vi "Live Imaging Window.vi"() -> ()   [LabVIEW 2020]
uses:
  Typedefs/Channel Selector.ctl
  SubVIs/Typedefs/Live window-ctrl refs.ctl
  Typedefs/Image display ref.ctl
  Typedefs/Left-Right enum.ctl
  Global Variables/General Globals.vi
  Globals/gl_Windows Ctrl refs.vi
panel:
  in  "Grid Visible":bool
  in  "Grid Lines":u32=2 min=2 max=10 step=1
  in  "Boolean":bool=TRUE
  in  "Pal":u32(ring) items=["Grayscale", "Binary", "Gradient", "Rainbow", "Temperature", "User Defined"]
  out "Running":bool
  out "Stop (ind)":bool
  in  "Snapshot Mode":bool
  out "Images received":i32
  out "Acq rate ind (Hz)":dbl format="Acquisition frame rate: %.1f fps"
  out "Refresh rate ind (Hz)":i32 format="Graph refresh rate: %.0f fps"
  in  "Right image intensity":cluster{i16, i16}(slide)={0, 2048} scale=0.0..4095.0
  in  "Right Image Palette":enum16{"Gray", "Red", "Green"}(ring) caption="Palette"
  in  "Right Channel":T1=enum."Green Channel"
  in  "Left image intensity":cluster{i16, i16}(slide)={0, 2048} scale=0.0..4095.0
  in  "Left Image Palette":enum16{"Gray", "Red", "Green"}(ring) caption="Palette"
  in  "Left Channel":T1
  in  "Sim":bool
  out "Right Image":T2(plugin-control)
  in  "Snapshot":bool
  out "Left Image":T2(plugin-control)
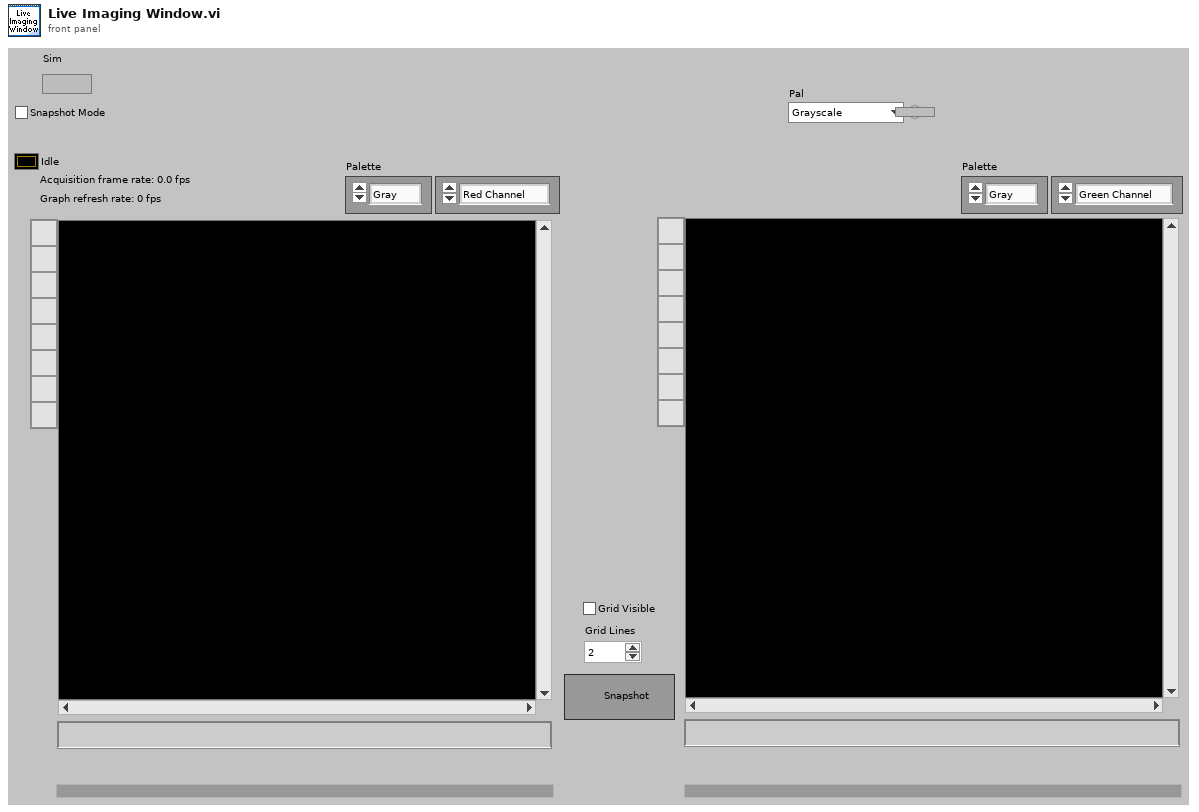
[diagram p1: front panel]
types:
  T1 = typedef "Channel Selector.ctl" = enum16{"Red Channel", "Green Channel", "Blended"}
  T2 = typedef "IMAQ Image.ctl" = refnum<image>
  T3 = typedef "Live window-ctrl refs.ctl" = cluster{"This VI":refnum<vi>, "Pane":refnum<vi>, "Show REF Image Left":refnum<vi>, "Show REF Image Right":refnum<vi>, "Snapshot":refnum<vi>, "Left Image Palette":refnum<vi>, "Right Image Palette":refnum<vi>, "Left Channel":refnum<vi>, "Right Channel":refnum<vi>, "Left image intensity":refnum<vi>, "Right image intensity":refnum<vi>, "Left Image Display":T4, "Right Image Display":T4, "Refresh rate ind (Hz)":refnum<vi>, "Acq rate ind (Hz)":refnum<vi>, "Stop (ind)":refnum<vi>}
  T4 = typedef "Image display ref.ctl" = refnum<vi>
  T5 = typedef "Live graph data queue ref.ctl" = refnum<queue>
  T6 = typedef "Left-Right enum.ctl" = enum16{"Right", "Left"}
  T7 = typedef "Live imaging queue element.ctl" = cluster{"Red channel":T2, "Green channel":T2, "Ref Red channel":T2, "Ref Green channel":T2, "Mov cor":bool}
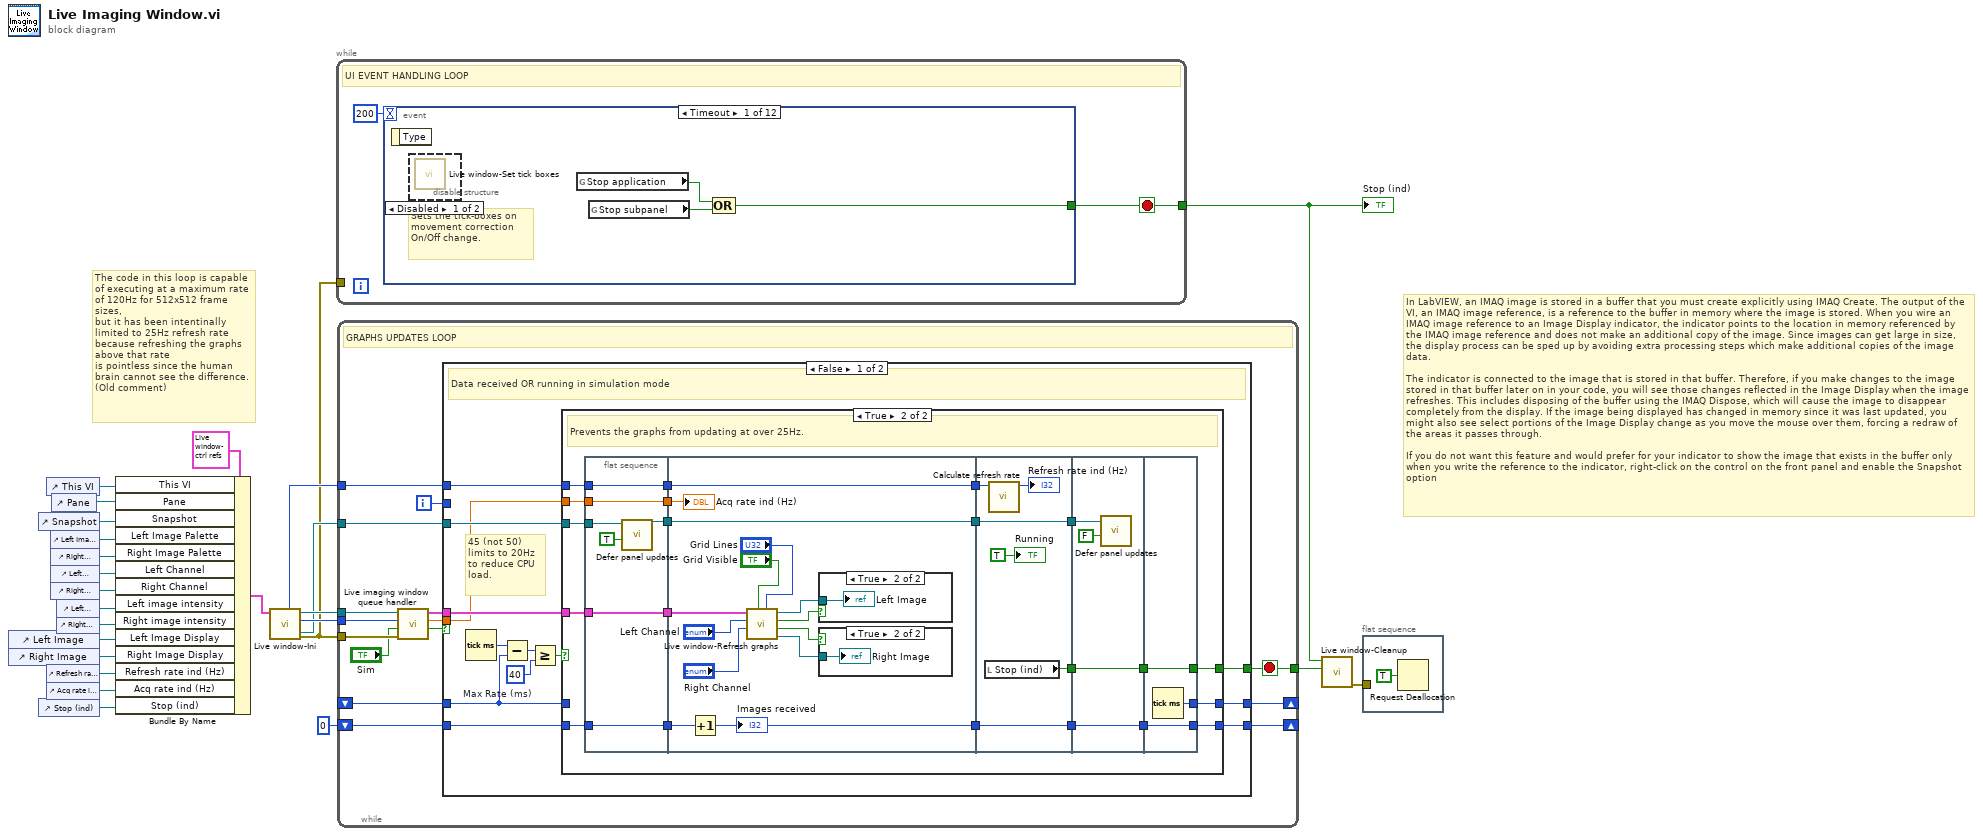
[diagram p0: block diagram]
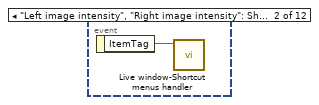
[diagram p3: hidden frame]
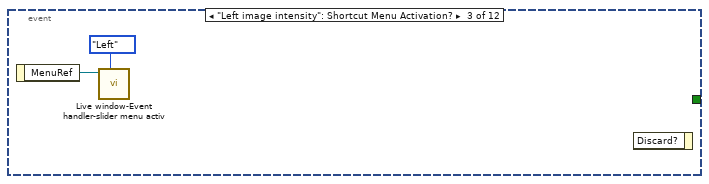
[diagram p4: hidden frame]
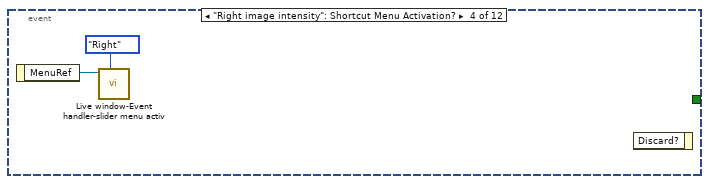
[diagram p5: hidden frame]
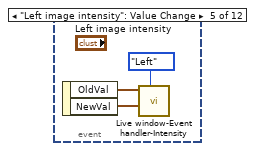
[diagram p6: hidden frame]
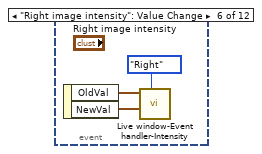
[diagram p7: hidden frame]
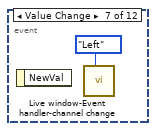
[diagram p8: hidden frame]
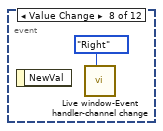
[diagram p9: hidden frame]
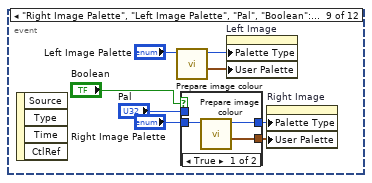
[diagram p10: hidden frame]
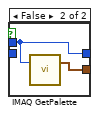
[diagram p11: hidden frame]
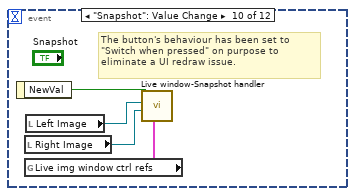
[diagram p12: hidden frame]
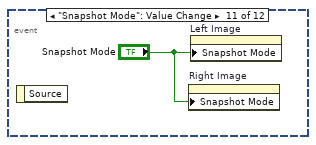
[diagram p13: hidden frame]
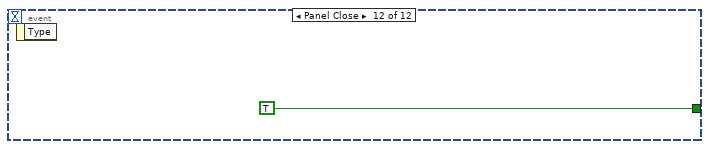
[diagram p14: hidden frame]
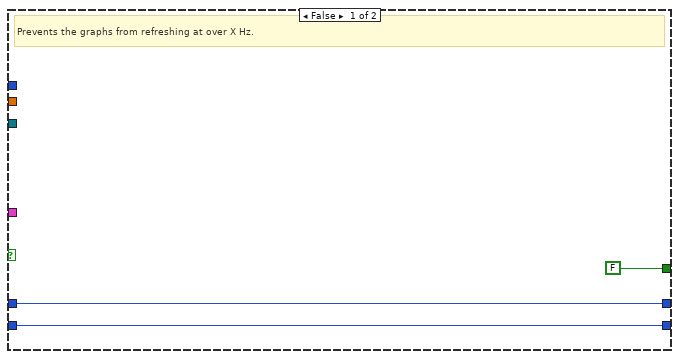
[diagram p15: hidden frame]
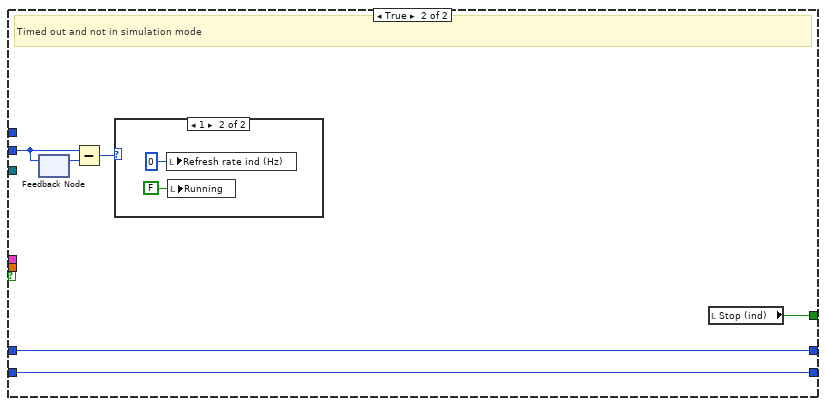
[diagram p18: hidden frame]
diagram:
  # "The code in this loop is capable of executing at a maximum rate of 120Hz for 512x512 frame sizes,\nbut it has been intentinally limited to 25Hz refresh rate because refreshing the graphs above that rate\nis pointless since the human brain cannot see the difference. (Old comment)"
  # "In LabVIEW, an IMAQ image is stored in a buffer that you must create explicitly using IMAQ Create. The output of the VI, an IMAQ image reference, is a reference to the buffer in memory where the image is stored. When you wire an IMAQ image reference to an Image Display indicator, the indicator points to the location in memory referenced by the IMAQ image reference and does not make an additional copy of the image. Since images can get large in size, the display process can be sped up by avoiding extra processing steps which make additional copies of the image data.\n\nThe indicator is connected to the image that is stored in that buffer. Therefore, if you make changes to the image stored in that buffer later on in your code, you will see those changes reflected in the Image Display when the image refreshes. This includes disposing of the buffer using the IMAQ Dispose, which will cause the image to disappear completely from the display. If the image being displayed has changed in memory since it was last updated, you might also see select portions of the Image Display change as you move the mouse over them, forcing a redraw of the areas it passes through.\n\nIf you do not want this feature and would prefer for your indicator to show the image that exists in the buffer only when you write the reference to the indicator, right-click on the control on the front panel and enable the Snapshot option"
  n1 = control-ref of="Left Image"() -> (w10:refnum<vi>)
  n2 = control-ref of="Right Image"() -> (w9:refnum<vi>)
  n3 = control-ref of="Snapshot"() -> (w13:refnum<vi>)
  n4 = control-ref of="Stop (ind)"() -> (w3:refnum<vi>)
  n5 = control-ref of="This VI"() -> (w15:refnum<vi>)
  n6 = control-ref of="Refresh rate ind (Hz)"() -> (w5:refnum<vi>)
  n7 = control-ref of="Acq rate ind (Hz)"() -> (w4:refnum<vi>)
  n8 = control-ref of="Left Image Palette"() -> (w21:refnum<vi>)
  n9 = control-ref of="Right Image Palette"() -> (w20:refnum<vi>)
  n10 = control-ref of="Left Channel"() -> (w19:refnum<vi>)
  n11 = control-ref of="Right Channel"() -> (w18:refnum<vi>)
  n12 = control-ref of="Pane"() -> (w7:refnum<vi>)
  n13 = control-ref of="Left image intensity"() -> (w17:refnum<vi>)
  n14 = control-ref of="Right image intensity"() -> (w16:refnum<vi>)
  n15 = Bundle By Name(cluster=T3 {"This VI"=refnum, "Pane"=refnum, "Show REF Image Left"=refnum, "Show REF Image Right"=refnum, "Snapshot"=refnum, "Left Image Palette"=refnum, "Right Image Palette"=refnum, "Left Channel"=refnum, "Right Channel"=refnum, "Left image intensity"=refnum, "Right image intensity"=refnum, "Left Image Display"=refnum, "Right Image Display"=refnum, "Refresh rate ind (Hz)"=refnum, "Acq rate ind (Hz)"=refnum, "Stop (ind)"=refnum} ("Live imaging window ctrl refs"), "This VI"=w15, "Pane"=w7, "Snapshot"=w13, "Left Image Palette"=w21, "Right Image Palette"=w20, "Left Channel"=w19, "Right Channel"=w18, "Left image intensity"=w17, "Right image intensity"=w16, "Left Image Display"=w10, "Right Image Display"=w9, "Refresh rate ind (Hz)"=w5, "Acq rate ind (Hz)"=w4, "Stop (ind)"=w3) -> (w11:T3)
  n16 = call "Live window-Ini.vi"("Live img window ctrl refs"=w11) -> ("error out"=w6:errorcluster, "Queue timeout"=w23:i32, "queue out"=w24:T5, "Front Panel"=w22:refnum<vi>, "Frame size"=w25:u16)  [unwired: 6 in]
  n17 = while {
    tunnel: [w26] -> w1
    tunnel: w6 -> [_]
    stop <- w26 stop-if-true
    # "UI EVENT HANDLING LOOP"
    n18 = event shown="[0] Timeout" {
      selector: _ -> [_ _ _ _ _ _ _ _ _ _ _ _]
      dyn-events: _ -> [_ _ _ _ _ _ _ _ _ _ _ _]
      timeout: 200 -> [_ _ _ _ _ _ _ _ _ _ _ _]
      tunnel: [w28 _ _ _ _ _ _ _ _ _ _ TRUE] -> w26
      event Timeout {
        # "Sets the tick-boxes on movement correction On/Off change."
        n19 = event-data() -> ()  [unwired: 1 in, 1 out]
        n20 = disable-structure shown="Disabled" {
          frame Disabled {
            n21 = call "Live window-Set tick boxes.vi"() -> ()  [unwired: 12 in]
          }
          frame Enabled {
          }
        }
        n22 = global read "General Globals.vi" "Stop application"() -> (w29:bool)
        n23 = global read "General Globals.vi" "Stop subpanel"() -> (w30:bool)
        n24 = Compound Arithmetic op=OR(w29, w30) -> (w28:bool)
      }
      event "Left image intensity", "Right image intensity": Shortcut Menu Selection (User) {
        n25 = event-data() -> ("ItemTag"=w31:string)  [unwired: 1 in]
        n26 = call "Live window-Shortcut menus handler.vi"("ItemTag"=w31) -> ()  [unwired: 11 in]
      }
      event "Left image intensity": Shortcut Menu Activation? {
        n27 = event-data() -> ("MenuRef"=w33:refnum<k9>)  [unwired: 1 in]
        n28 = call "Live window-Event handler-slider menu activ.vi"("Left/Right"=Left-Right_enum."Left", "Image intensity slider Menu"=w33) -> ()  [unwired: 10 in]
        n29 = event-data() -> ()  [unwired: 2 in, 1 out]
      }
      event "Right image intensity": Shortcut Menu Activation? {
        n30 = event-data() -> ("MenuRef"=w34:refnum<k9>)  [unwired: 1 in]
        n31 = call "Live window-Event handler-slider menu activ.vi"("Left/Right"=Left-Right_enum."Right", "Image intensity slider Menu"=w34) -> ()  [unwired: 10 in]
        n32 = event-data() -> ()  [unwired: 2 in, 1 out]
      }
      event "Left image intensity": Value Change {
        n33 = event-data() -> ("OldVal"=w38:cluster{i16, i16}, "NewVal"=w37:cluster{i16, i16})  [unwired: 1 in]
        n34 = call "Live window-Event handler-Intensity.vi"("Which image display?"=Left-Right_enum."Left", "NewVal"=w37, "OldVal"=w38) -> ()  [unwired: 9 in]
      }
      event "Right image intensity": Value Change {
        n35 = event-data() -> ("OldVal"=w40:cluster{i16, i16}, "NewVal"=w41:cluster{i16, i16})  [unwired: 1 in]
        n36 = call "Live window-Event handler-Intensity.vi"("Which image display?"=Left-Right_enum."Right", "NewVal"=w41, "OldVal"=w40) -> ()  [unwired: 9 in]
      }
      event Value Change {
        n37 = event-data() -> ()  [unwired: 1 in, 1 out]
        n38 = call "Live window-Event handler-channel change.vi"("Left/Right"=Left-Right_enum."Left") -> ()  [unwired: 10 in, 1 out]
      }
      event Value Change {
        n39 = event-data() -> ()  [unwired: 1 in, 1 out]
        n40 = call "Live window-Event handler-channel change.vi"("Left/Right"=Left-Right_enum."Right") -> ()  [unwired: 10 in, 1 out]
      }
      event "Right Image Palette", "Left Image Palette", "Pal", "Boolean": Value Change {
        n41 = event-data() -> ()  [unwired: 1 in, 4 out]
        n42 = call "Prepare image colour.vi"("Left Image Palette"="Left Image Palette") -> ("Color Palette"=w49:cluster{"Red":u8, "Green":u8, "Blue":u8}[], "Palette Type"=w51:u32)  [unwired: 8 in, 1 out]
        n43 = case shown="True" "Boolean" {
          tunnel: [w54 w56] -> w48
          tunnel: "Right Image Palette" -> [w53 _]
          tunnel: [w52 w55] -> w46
          tunnel: "Pal" -> [_ w55]
          frame True {
            n44 = call "Prepare image colour.vi"("Left Image Palette"=w53) -> ("Color Palette"=w54:cluster{"Red":u8, "Green":u8, "Blue":u8}[], "Palette Type"=w52:u32)  [unwired: 8 in, 1 out]
          }
          frame False {
            n45 = call "IMAQ GetPalette"("Palette Number (gray)"=w55) -> ("Color Palette"=w56:cluster{"Red":u8, "Green":u8, "Blue":u8}[])  [unwired: 4 in, 1 out]
          }
        }
        n46 = property on="Left Image" class="ImageControl"("Palette Type"=w51, "User Palette"=w49) -> ()  [unwired: 2 in, 2 out]
        n47 = property on="Right Image" class="ImageControl"("Palette Type"=w46, "User Palette"=w48) -> ()  [unwired: 2 in, 2 out]
      }
      event "Snapshot": Value Change {
        # "The button's behaviour has been set to \"Switch when pressed\" on purpose to eliminate a UI redraw issue."
        n48 = event-data() -> ("NewVal"=w60:bool)  [unwired: 1 in]
        n49 = local read "Right Image"() -> (w58:T2)
        n50 = global read "gl_Windows Ctrl refs.vi" "Live img window ctrl refs"() -> (w57:T3)
        n51 = local read "Left Image"() -> (w59:T2)
        n52 = call "Live window-Snapshot handler.vi"("Window ctrl refs"=w57, "Right image"=w58, "Left image"=w59, "Snapshot:NewVal"=w60) -> ()  [unwired: 8 in]
      }
      event "Snapshot Mode": Value Change {
        n53 = event-data() -> ()  [unwired: 1 in, 1 out]
        n54 = property on="Right Image" class="ImageControl"("Snapshot Mode"="Snapshot Mode") -> ()  [unwired: 2 in, 2 out]
        n55 = property on="Left Image" class="ImageControl"("Snapshot Mode"="Snapshot Mode") -> ()  [unwired: 2 in, 2 out]
      }
      event Panel Close {
        n56 = event-data() -> ()  [unwired: 1 in, 1 out]
      }
    }
  }
  "Stop (ind)" <- w1
  n57 = while {
    tunnel: w24 -> [w77]
    tunnel: w6 -> [w76]
    tunnel: w23 -> [w74]
    tunnel: [w64] -> w12
    shift-right: [w72] -> _
    shift-left: 0 -> [w68]
    tunnel: w25 -> [w71]
    shift-right: [w70] -> _
    shift-left: _ -> [w69]
    tunnel: w22 -> [w66]
    i -> [w63]
    stop <- w64 stop-if-true
    # "GRAPHS UPDATES LOOP"
    n58 = call "Live imaging window queue handler.vi"("error in (no error)"=w76, "Sim"="Sim", "timeout in ms"=w74, "Queue in"=w77) -> ("timed out?"=w67:bool, "Frame rate (Hz)"=w65:dbl, "Element to queue"=w75:T7)  [unwired: 5 in]
    n59 = case shown="False" w67 {
      tunnel: w75 -> [w90 _]
      tunnel: [w89 w156] -> w72
      tunnel: w68 -> [w82 w156]
      tunnel: w71 -> [w83 _]
      tunnel: [w88 w155] -> w70
      tunnel: w69 -> [w85 w155]
      tunnel: w66 -> [w81 _]
      tunnel: w65 -> [w80 _]
      tunnel: [w79 w154] -> w64
      tunnel: w63 -> [_ w152]
      frame False {
        w78 = u32 40  # Max Rate (ms)
        # "45 (not 50)\nlimits to 20Hz\nto reduce CPU\nload."
        # "Data received OR running in simulation mode"
        n60 = Tick Count (ms)() -> (millisecond timer value=w87:u32)
        n61 = Subtract(x=w87, y=w85) -> (x-y=w86:u32)
        n62 = Greater Or Equal?(x=w86, y=w78) -> (x >= y?=w84:bool)
        n63 = case shown="True" w84 {
          tunnel: w90 -> [_ w114]
          tunnel: [w93 w113] -> w89
          tunnel: [w92 w112] -> w88
          tunnel: w82 -> [w93 w111]
          tunnel: w85 -> [w92 _]
          tunnel: w83 -> [_ w110]
          tunnel: w81 -> [_ w109]
          tunnel: w80 -> [_ w103]
          tunnel: [FALSE w96] -> w79
          frame False {
            # "Prevents the graphs from refreshing at over X Hz."
          }
          frame True {
            # "Prevents the graphs from updating at over 25Hz."
            n64 = flat-sequence {
              tunnel: w103 -> [w118]
              tunnel: w109 -> [w117]
              tunnel: w110 -> [w119]
              tunnel: w114 -> [w120]
              tunnel: w111 -> [w121]
              tunnel: [w121] -> w102
              tunnel: [w120] -> w101
              tunnel: [w119] -> w100
              tunnel: [w116] -> w99
              tunnel: [w118] -> w98
              tunnel: [w129] -> w108
              tunnel: [w135] -> w106
              tunnel: [w127] -> w105
              tunnel: w102 -> [w130]
              tunnel: w101 -> [w128]
              tunnel: w100 -> [w135]
              tunnel: w99 -> [w127]
              tunnel: w98 -> [w126]
              tunnel: w108 -> [w143]
              tunnel: [w143] -> w107
              tunnel: w106 -> [w140]
              tunnel: w105 -> [w142]
              tunnel: [w142] -> w104
              tunnel: [w138] -> w94
              tunnel: w107 -> [w147]
              tunnel: w104 -> [w146]
              tunnel: [w147] -> w97
              tunnel: [w145] -> w95
              tunnel: w94 -> [w145]
              tunnel: [w149] -> w112
              tunnel: [w150] -> w113
              tunnel: w97 -> [w150]
              tunnel: [w148] -> w96
              tunnel: w95 -> [w148]
              frame #0 {
                n65 = call "Defer panel updates.vi"("Defer Panel Updates"=TRUE, "Panel in"=w117) -> ("Panel out"=w116:refnum<vi>)  [unwired: 9 in]
              }
              frame #1 {
                n66 = Increment(x=w130) -> (x+1=w129:i32)
                "Images received" <- w129
                n67 = call "Live window-Refresh graphs.vi"("Grid Lines"="Grid Lines", "Visible(Grid)"="Grid Visible", "Right Channel"="Right Channel", "Left Channel"="Left Channel", "Element to queue"=w128) -> ("Right image"=w133:T2, "Enable right image"=w131:bool, "Enable left image"=w132:bool, "Left image"=w134:T2)  [unwired: 3 in]
                n68 = case shown="True" w132 {
                  tunnel: w134 -> [_ w137]
                  frame False {
                  }
                  frame True {
                    "Left Image" <- w137
                  }
                }
                n69 = case shown="True" w131 {
                  tunnel: w133 -> [_ w136]
                  frame False {
                  }
                  frame True {
                    "Right Image" <- w136
                  }
                }
                "Acq rate ind (Hz)" <- w126
              }
              frame #2 {
                n70 = local read "Stop (ind)"() -> (w138:bool)
                n71 = call "Calculate refresh rate.vi"("Frame size"=w140) -> ("Refresh rate (Hz)"=→"Refresh rate ind (Hz)":i32)  [unwired: 9 in, 1 out]
                "Running" <- TRUE ("Running")
              }
              frame #3 {
                n72 = call "Defer panel updates.vi"("Defer Panel Updates"=FALSE, "Panel in"=w146) -> ()  [unwired: 9 in, 1 out]
              }
              frame #4 {
                n73 = Tick Count (ms)() -> (millisecond timer value=w149:u32)
              }
            }
          }
        }
      }
      frame True {
        # "Timed out and not in simulation mode"
        n74 = feedback-in #1(w152) -> ()
        n75 = feedback #1() -> (w153:i32)  [unwired: 1 in]
        n76 = Subtract(x=w152, y=w153) -> (x-y=w151:i32)
        n77 = case shown="1" w151 {
          frame Default {
          }
          frame 1 {
            n78 = local write "Refresh rate ind (Hz)"(0 ("Refresh rate ind (Hz)")) -> ()
            n79 = local write "Running"(FALSE ("Running")) -> ()
          }
        }
        n80 = local read "Stop (ind)"() -> (w154:bool)
      }
    }
  }
  n81 = call "Live window-Cleanup.vi"("Stop"=w12, "Boolean"=w1) -> ("error out"=w2:errorcluster)  [unwired: 9 in]
  n82 = flat-sequence {
    tunnel: w2 -> [_]
    frame #0 {
      n83 = Request Deallocation(TRUE ("flag")) -> ()
    }
  }
